vi "wfm_feature update_xygraph_auto_scale.vi"(8 "error in (no error)":errorcluster, 11 "wfm_feature in":refnum<class "wfm_feature.lvclass">) -> (0 "error out":errorcluster, 3 "wfm_feature out":refnum<class "wfm_feature.lvclass">)   [LabVIEW 2018, in "wfm_feature.lvclass"]
uses:
  wfm_feature.lvclass
  wfm_feature.lvclass/wfm_feature.ctl
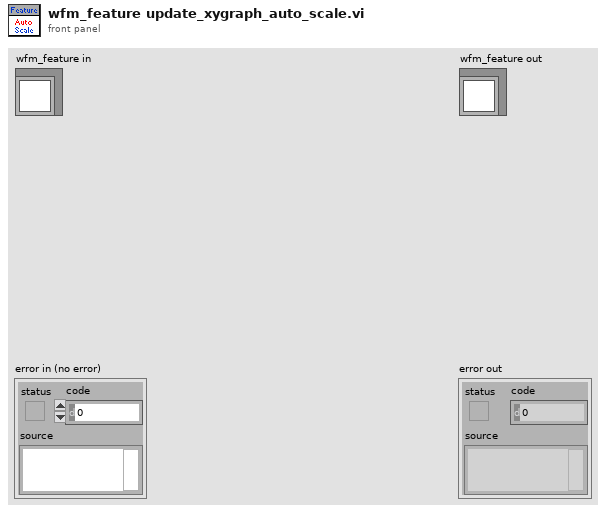
[diagram p1: front panel]
types:
  T1 = typedef "LVRangeTypeDef.ctl" = cluster{"Minimum":dbl, "Maximum":dbl, "Increment":dbl, "Minor Increment":dbl, "Start":dbl}
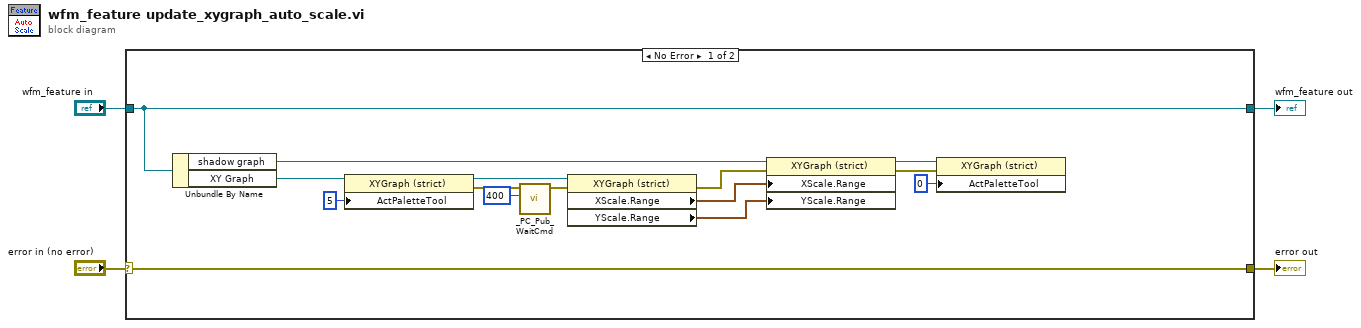
[diagram p0: block diagram]
diagram:
  n1 = case shown="No Error" "error in (no error)" {
    selector: "error in (no error)" -> [w19 w21]
    tunnel: [w19 w21] -> w3
    tunnel: [w18 w20] -> w1
    tunnel: "wfm_feature in" -> [w18 w20]
    frame No Error {
      n2 = Unbundle By Name(w18) -> ("shadow graph"=w15:refnum<vi>, "XY Graph"=w17:refnum<vi>)
      n3 = property class="XYGraph (strict)"(reference=w17, "ActPaletteTool"=5 ("Palette:Active Tool")) -> (reference out=w9:refnum<vi>, error out=w11:errorcluster)  [unwired: 1 in]
      n4 = call "_PC_Pub_WaitCmd.vi"("milliseconds to wait"=u32 400, "error in (no error)"=w11) -> ("error out"=w8:errorcluster)  [unwired: 9 in]
      n5 = property class="XYGraph (strict)"(reference=w9, error in=w8) -> (error out=w12:errorcluster, "XScale.Range"=w14:T1, "YScale.Range"=w13:T1)  [unwired: 1 out]
      n6 = property class="XYGraph (strict)"(reference=w15, error in=w12, "XScale.Range"=w14, "YScale.Range"=w13) -> (reference out=w6:refnum<vi>, error out=w5:errorcluster)
      n7 = property class="XYGraph (strict)"(reference=w6, error in=w5, "ActPaletteTool"=0 ("Palette:Active Tool")) -> ()  [unwired: 2 out]
    }
    frame Error {
    }
  }
  "error out" <- w3
  "wfm_feature out" <- w1
